vi "Configure Constant Resistance.vi"(0 "VISA resource name":refnum<visa-resource-name>, 5 "CR Resistance (1)":dbl=1.0 min=0.0 max=7500.0 step=1.0 format="%#.4g", 7 "Voltage Maximum (120.000)":dbl=120.0 min=0.0 max=520.0 step=1.0 format="%.3f", 9 "Voltage Minimum (0)":dbl min=0.0 max=520.0 step=1.0 format="%.3f", 11 "error in (no error)":errorcluster, 12 "Enable CR LED Mode (F: False)":bool, 13 "LED Forward Voltage (0)":dbl min=0.0 max=520.0 step=1.0 format="%.3f") -> (4 "VISA resource name out":refnum<visa-resource-name>, 15 "error out":errorcluster)   [LabVIEW 2018, in "BK Precision 8600 Series.lvlib"]
doc: "Configures the resistance for constant resistance (CR) operation and configures CR LED mode."
uses:
  <instrlib>/BK Precision 8600 Series/BK Precision 8600 Series.lvlib
panel:
  # "V"
  # "V"
  # "V"
  # "Ohm"
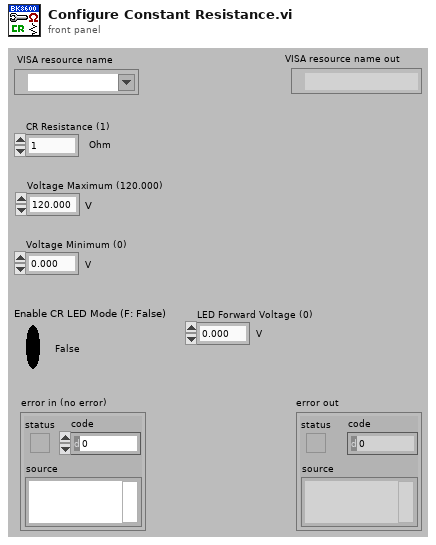
[diagram p1: front panel]
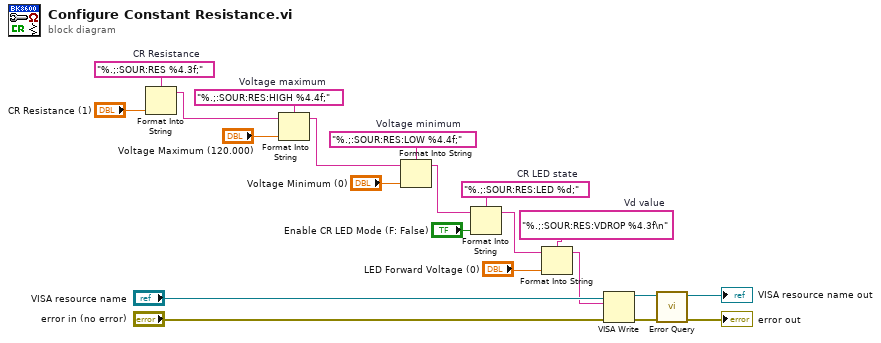
[diagram p0: block diagram]
diagram:
  w1 = "%.;:SOUR:RES:VDROP %4.3f\n"  # Vd value
  w5 = "%.;:SOUR:RES:LED %d;"  # CR LED state
  w15 = "%.;:SOUR:RES:LOW %4.4f;"  # Voltage minimum
  w14 = "%.;:SOUR:RES:HIGH %4.4f;"  # Voltage maximum
  w19 = "%.;:SOUR:RES %4.3f;"  # CR Resistance
  n1 = Format Into String(format string=w19, "CR Resistance (1)") -> (resulting string=w10:string)  [unwired: 2 in, 1 out]
  n2 = Format Into String(format string=w14, initial string=w10, "Voltage Maximum (120.000)") -> (resulting string=w12:string)  [unwired: 1 in, 1 out]
  n3 = Format Into String(format string=w15, initial string=w12, "Voltage Minimum (0)") -> (resulting string=w6:string)  [unwired: 1 in, 1 out]
  n4 = Format Into String(format string=w5, initial string=w6, "Enable CR LED Mode (F: False)") -> (resulting string=w3:string)  [unwired: 1 in, 1 out]
  n5 = Format Into String(format string=w1, initial string=w3, "LED Forward Voltage (0)") -> (resulting string=w2:string)  [unwired: 1 in, 1 out]
  n6 = VISA Write(VISA resource name="VISA resource name", write buffer=w2, error in (no error)="error in (no error)") -> (VISA resource name out=w17:refnum<visa-resource-name>, error out=w18:errorcluster)  [unwired: 1 out]
  n7 = call <instrlib>:"Error Query.vi"("error in (no error)"=w18, "VISA resource name"=w17) -> ("error out"=→"error out":errorcluster, "VISA resource name out"=→"VISA resource name out":refnum<visa-resource-name>)  [unwired: 6 in, 2 out]
